vi "LiveAcquireold.vi"() -> ()   [LabVIEW 2015]
uses:
  <userlib>/atmcd64d.llb/AcquisitionMode_mode typedef.ctl
  NIDAQControls/StateGlobals.vi
  AcquisitionGlobals.vi
  NIDAQControls/NIDAQGlobals.vi
  LiveImage_Global.vi
panel:
  out "size(s)":i32
  out "xpixels 2":i32
  out "ypixels 2":i32
  out "Acquire Time":dbl
  out "Wait Time":dbl
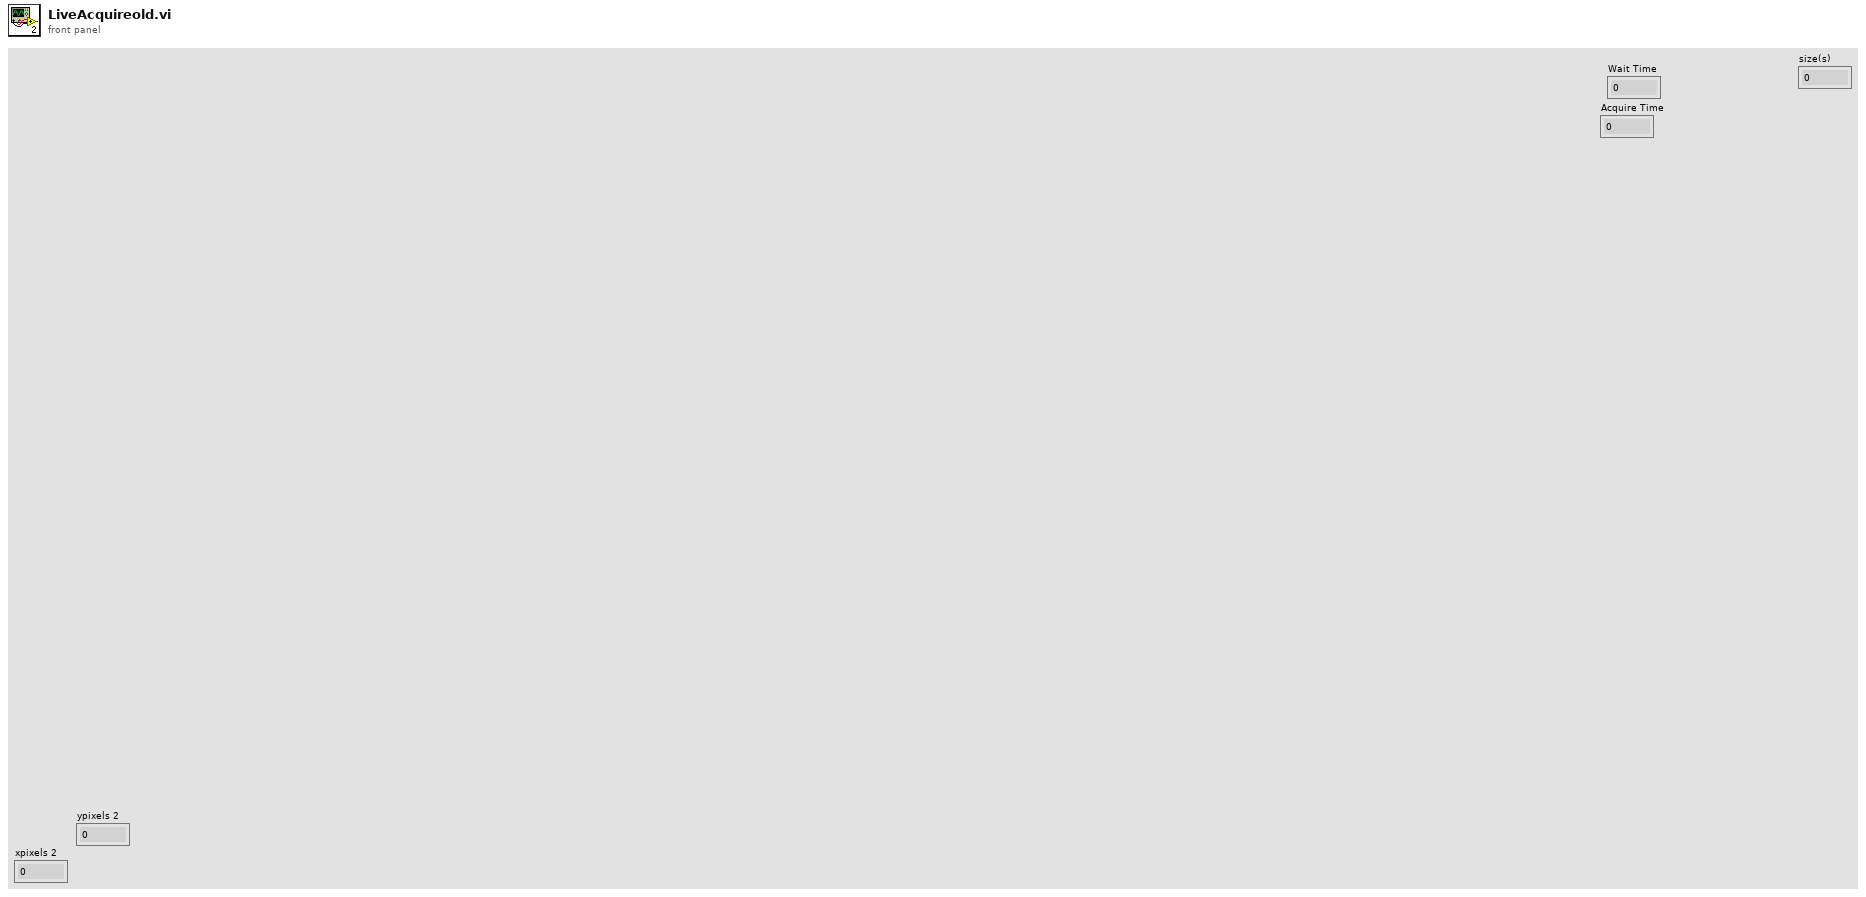
[diagram p1: front panel]
types:
  T1 = cluster{"Start or New Parameters?":bool, "Laser Mode":string, "Piezo Mode":string, "Begin Or End Acquisition":string, "Acquisition Time":dbl}
  T2 = typedef "AcquisitionMode_mode typedef.ctl" = enum16{"Reserved (0)", "Single Scan", "Accumulate", "Kinetics", "Fast Kinetics", "Run Till Abort", "Reserved (6)", "Reserved (7)", "Reserved (8)", "Time Delayed Integration"}
  T3 = typedef "Rendezvous RefNum" = refnum<k1>
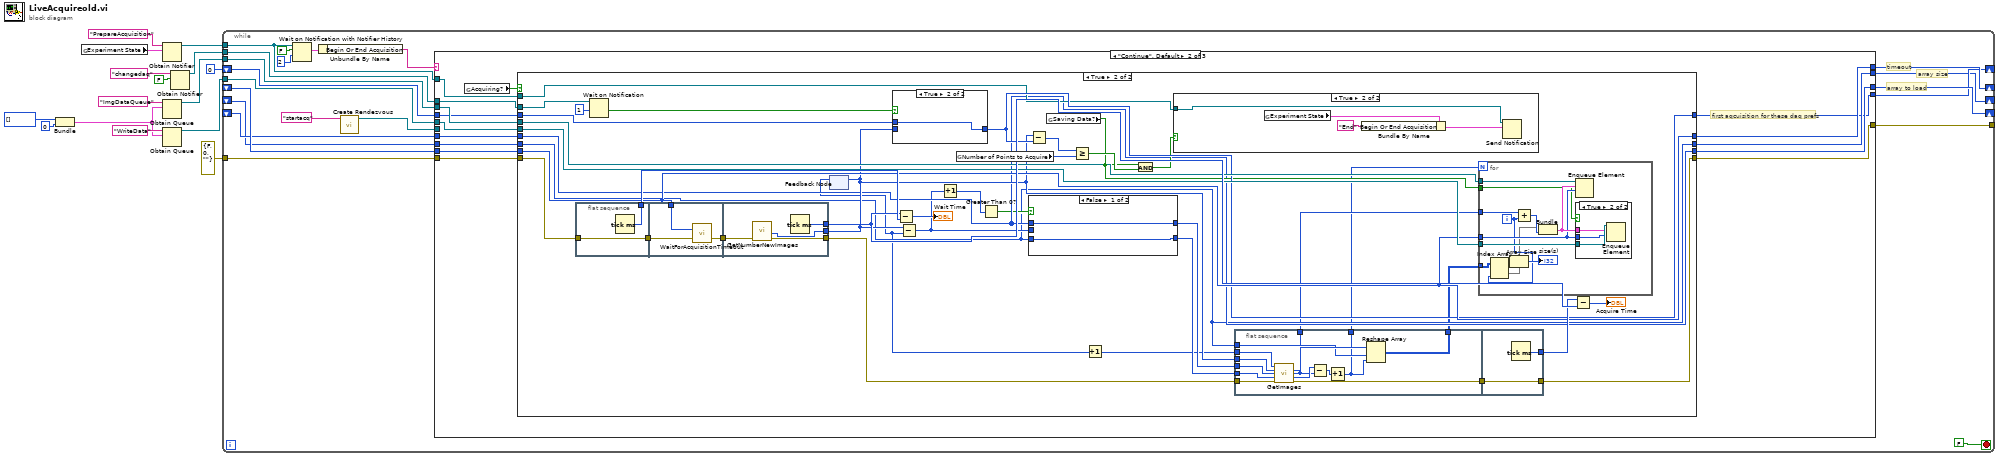
[diagram p0: block diagram]
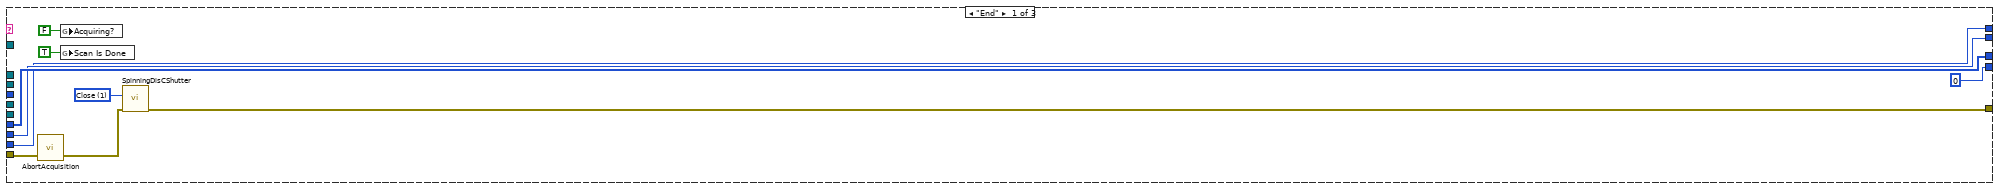
[diagram p2: hidden frame]
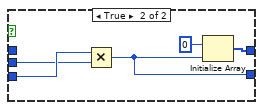
[diagram p5: hidden frame]
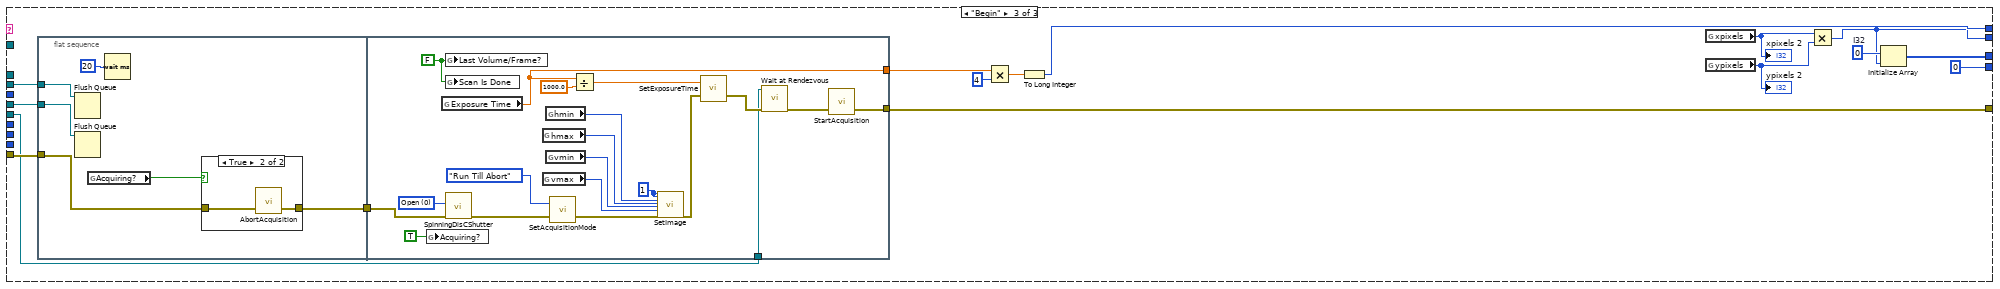
[diagram p8: hidden frame]
diagram:
  n1 = Bundle(u16[] [], 0) -> (w8:cluster{u16[], i32})  [unwired: 1 in]
  n2 = global read "StateGlobals.vi" "Experiment State"() -> (w1:T1)
  n3 = Obtain Notifier(name (unnamed)="PrepareAcquisition", notification data type=w1) -> (notifier out=w13:refnum<notifier>)  [unwired: 2 in, 2 out]
  n4 = Obtain Queue(name (unnamed)="ImgDataQueue", element data type=w8) -> (queue out=w6:refnum<queue>)  [unwired: 3 in, 2 out]
  n5 = Obtain Queue(name (unnamed)="WriteData", element data type=w8) -> (queue out=w7:refnum<queue>)  [unwired: 3 in, 2 out]
  n6 = Obtain Notifier(name (unnamed)="changedaq", notification data type=FALSE) -> (notifier out=w2:refnum<notifier>)  [unwired: 2 in, 2 out]
  n7 = while {
    tunnel: w13 -> [w17]
    shift-right: [w33] -> _
    shift-left: _ -> [w29]
    shift-right: [w32] -> _
    shift-left: _ -> [w28]
    shift-right: [w16] -> _
    shift-left: _ -> [w24]
    tunnel: w7 -> [w27]
    tunnel: w6 -> [w26]
    tunnel: errorcluster {"status"=FALSE, "code"=0, "source"=""} ("error out") -> [w31]
    tunnel: [w30] -> _
    shift-right: [w19] -> _
    shift-left: 0 -> [w20]
    tunnel: w2 -> [w18]
    stop <- FALSE stop-if-true
    # "array size"
    # "timeout"
    # "array to load"
    n8 = Wait on Notification with Notifier History(0:w17, 1:FALSE ("ignore previous (F)"), 2:2 ("timeout in ms (-1)")) -> (9:w35:T1)  [unwired: 1 in, 3 out]
    n9 = Unbundle By Name(w35) -> ("Begin Or End Acquisition"=w34:string)
    n10 = call <vilib>:"Create Rendezvous.vi"("name (unnamed)"="startacq") -> ("rendezvous"=w22:T3)  [unwired: 4 in, 2 out]
    n11 = case shown="\"Continue\", Default" w34 {
      tunnel: [w38 w54 w166] -> w33
      tunnel: [w40 w55 w165] -> w32
      tunnel: [w39 w53 w164] -> w16
      tunnel: w31 -> [w42 w59 w163]
      tunnel: [w41 w56 w162] -> w30
      tunnel: w29 -> [w38 w60 _]
      tunnel: w28 -> [w40 w58 _]
      tunnel: w24 -> [w39 w57 _]
      tunnel: w27 -> [_ w52 w157]
      tunnel: w26 -> [_ w51 w158]
      tunnel: w22 -> [_ _ w159]
      tunnel: w20 -> [_ w50 _]
      tunnel: [0 ("last") w48 0 ("last")] -> w19
      tunnel: w18 -> [_ w49 _]
      tunnel: w17 -> [_ w47 _]
      frame "End" {
        w44 = u16 1 items=["Open", "Close"] ("Ring")
        n12 = call <userlib>:"AbortAcquisition.vi"("error in (no error)"=w42) -> ("error out"=w43:errorcluster)  [unwired: 1 in, 1 out]
        n13 = global write "AcquisitionGlobals.vi" "Acquiring?"(FALSE) -> ()
        n14 = global write "NIDAQGlobals.vi" "Scan Is Done"(TRUE ("Last Volume/Frame?")) -> ()
        n15 = call "SpinningDisCShutter.vi"("error in (no error)"=w43, "Ring"=w44) -> ("error out"=w41:errorcluster)  [unwired: 9 in]
      }
      frame "Continue", Default {
        # "first aqcuisition for these daq prefs"
        n16 = global read "AcquisitionGlobals.vi" "Acquiring?"() -> (w61:bool)
        n17 = case shown="True" w61 {
          tunnel: w60 -> [w63 w91]
          tunnel: w59 -> [w65 w102]
          tunnel: w58 -> [w64 w78]
          tunnel: w57 -> [w66 w73]
          tunnel: [w65 w94] -> w56
          tunnel: [w64 w78] -> w55
          tunnel: [w63 w91] -> w54
          tunnel: [w66 w73] -> w53
          tunnel: w52 -> [_ w92]
          tunnel: w51 -> [_ w93]
          tunnel: w50 -> [w62 w88]
          tunnel: [w62 w87] -> w48
          tunnel: w49 -> [_ w90]
          tunnel: w47 -> [_ w82]
          frame False {
          }
          frame True {
            n18 = flat-sequence {
              tunnel: w102 -> [w148]
              tunnel: [w148] -> w104
              tunnel: [w147] -> w99
              tunnel: w104 -> [w151]
              tunnel: [w150] -> w103
              tunnel: w91 -> [w149]
              tunnel: [w153] -> w100
              tunnel: w103 -> [w154]
              tunnel: [w155] -> w97
              tunnel: [w152] -> w79
              frame #0 {
                n19 = Tick Count (ms)() -> (millisecond timer value=w147:u32)
              }
              frame #1 {
                n20 = call <userlib>:"WaitForAcquisitionTimeout.vi"("error in (no error)"=w151, "iTimeOutMs"=w149) -> ("error out"=w150:errorcluster)  [unwired: 1 out]
              }
              frame #2 {
                n21 = call <userlib>:"GetNumberNewImages.vi"("error in (no error)"=w154) -> ("error out"=w153:errorcluster, "last"=w152:i32)  [unwired: 3 in, 2 out]
                n22 = Tick Count (ms)() -> (millisecond timer value=w155:u32)
              }
            }
            n23 = Wait on Notification(notifier=w90, timeout in ms (-1)=1) -> (timed out?=w89:bool)  [unwired: 2 in, 3 out]
            n24 = feedback-in #1(w79) -> ()
            n25 = feedback #1() -> (w68:i32)  [unwired: 1 in]
            n26 = case shown="True" w89 {
              tunnel: w88 -> [_ w131]
              tunnel: w79 -> [w130 _]
              tunnel: [w130 w131] -> w87
              frame False {
              }
              frame True {
              }
            }
            n27 = Subtract(x=w97, y=w99) -> (x-y=→"Wait Time":u32)
            n28 = Subtract(x=w79, y=w68) -> (x-y=w74:i32)
            n29 = Increment(x=w74) -> (x+1=w70:i32)
            n30 = global read "StateGlobals.vi" "Number of Points to Acquire"() -> (w85:i32)
            n31 = Greater Than 0?(x=w70) -> (x > 0?=w75:bool)
            n32 = case shown="False" w75 {
              tunnel: w73 -> [w119 w124]
              tunnel: w78 -> [w120 _]
              tunnel: [w120 w122] -> w77
              tunnel: [w119 w121] -> w76
              tunnel: w74 -> [_ w123]
              frame False {
              }
              frame True {
                n33 = Multiply(x=w124, y=w123) -> (x*y=w121:i32)
                n34 = Initialize Array(u16 0 ("element"), w121) -> (w122:u16[])
              }
            }
            n35 = Subtract(x=w79, y=w87) -> (x-y=w80:i32)
            n36 = global read "AcquisitionGlobals.vi" "Saving Data?"() -> (w83:bool)
            n37 = Greater Or Equal?(x=w80, y=w85) -> (x >= y?=w84:bool)
            n38 = Increment(x=w68) -> (x+1=w69:i32)
            n39 = And(x=w83, y=w84) -> (x .and. y?=w81:bool)
            n40 = case shown="True" w81 {
              tunnel: w82 -> [_ w129]
              frame False {
              }
              frame True {
                n41 = global read "StateGlobals.vi" "Experiment State"() -> (w128:T1)
                n42 = Bundle By Name(cluster=w128, "Begin Or End Acquisition"="End") -> (w126:T1)
                n43 = Send Notification(notification=w126, notifier=w129) -> ()  [unwired: 1 in, 2 out]
              }
            }
            n44 = flat-sequence {
              tunnel: w77 -> [w140]
              tunnel: [w144] -> w101
              tunnel: w100 -> [w143]
              tunnel: w79 -> [w142]
              tunnel: w69 -> [w141]
              tunnel: w76 -> [w139]
              tunnel: w73 -> [w136]
              tunnel: [w135] -> w72
              tunnel: [w134] -> w71
              tunnel: [w132] -> w67
              tunnel: [w146] -> w94
              tunnel: w101 -> [w146]
              tunnel: [w145] -> w96
              frame #0 {
                n45 = call <userlib>:"GetImages.vi"("first"=w141, "last"=w142, "array"=w140, "size"=w139, "error in (no error)"=w143) -> ("array"=w138:i32[], "validfirst"=w134:i32, "validlast"=w137:i32, "error out"=w144:errorcluster)  [unwired: 6 in, 1 out]
                n46 = Subtract(x=w137, y=w134) -> (x-y=w133:i32)
                n47 = Increment(x=w133) -> (x+1=w132:i32)
                n48 = Reshape Array(w138, w136, w132) -> (w135:i32[][])
              }
              frame #1 {
                n49 = Tick Count (ms)() -> (millisecond timer value=w145:u32)
              }
            }
            n50 = for {
              N: w67 -> [_]
              tunnel: w93 -> [w114]
              tunnel: w92 -> [w113]
              tunnel: w91 -> [w112]
              tunnel: w83 -> [w111]
              tunnel: w72 -> [w107]
              tunnel: w71 -> [w110]
              i -> [w106]
              n51 = Index Array(array=w107, index (col)=w106) -> (element=w105:i32[])  [unwired: 1 in]
              n52 = Array Size(array=w105) -> (size(s)=→"size(s)":i32)
              n53 = Add(x=w110, y=w106) -> (x+y=w109:i32)
              n54 = Bundle("array"=w105, w109) -> (w115:cluster{"array":i32[], i32})  [unwired: 1 in]
              n55 = Enqueue Element(queue=w114, element=w115, timeout in ms (-1)=w112) -> ()  [unwired: 1 in, 3 out]
              n56 = case shown="True" w111 {
                tunnel: w113 -> [_ w118]
                tunnel: w112 -> [_ w117]
                tunnel: w115 -> [_ w116]
                frame False {
                }
                frame True {
                  n57 = Enqueue Element(queue=w118, element=w116, timeout in ms (-1)=w117) -> ()  [unwired: 1 in, 3 out]
                }
              }
            }
            n58 = Subtract(x=w96, y=w97) -> (x-y=→"Acquire Time":u32)
          }
        }
      }
      frame "Begin" {
        w169 = u16 0  # I32
        n59 = flat-sequence {
          tunnel: w163 -> [w177]
          tunnel: [w176] -> w161
          tunnel: w158 -> [w174]
          tunnel: w157 -> [w173]
          tunnel: [w196] -> w162
          tunnel: w161 -> [w197]
          tunnel: [w184] -> w160
          tunnel: w159 -> [w181]
          frame #0 {
            n60 = Flush Queue(queue=w174) -> ()  [unwired: 1 in, 3 out]
            n61 = Flush Queue(queue=w173) -> ()  [unwired: 1 in, 3 out]
            n62 = global read "AcquisitionGlobals.vi" "Acquiring?"() -> (w175:bool)
            n63 = Wait (ms)(milliseconds to wait=u32 20) -> ()  [unwired: 1 out]
            n64 = case shown="True" w175 {
              tunnel: w177 -> [w178 w180]
              tunnel: [w178 w179] -> w176
              frame False {
              }
              frame True {
                n65 = call <userlib>:"AbortAcquisition.vi"("error in (no error)"=w180) -> ("error out"=w179:errorcluster)  [unwired: 1 in, 1 out]
              }
            }
          }
          frame #1 {
            w193 = 1
            w195 = FALSE ("Last Volume/Frame?")
            w199 = u16 0 items=["Open", "Close"] ("Ring")
            n66 = global write "AcquisitionGlobals.vi" "Acquiring?"(TRUE) -> ()
            n67 = global read "LiveImage_Global.vi" "Exposure Time"() -> (w184:dbl)
            n68 = global write "NIDAQGlobals.vi" "Last Volume/Frame?"(w195) -> ()
            n69 = global write "NIDAQGlobals.vi" "Scan Is Done"(w195) -> ()
            n70 = call "SpinningDisCShutter.vi"("error in (no error)"=w197, "Ring"=w199) -> ("error out"=w198:errorcluster)  [unwired: 9 in]
            n71 = global read "LiveImage_Global.vi" "hmax"() -> (w191:i32)
            n72 = global read "LiveImage_Global.vi" "vmax"() -> (w189:i32)
            n73 = global read "LiveImage_Global.vi" "hmin"() -> (w192:i32)
            n74 = global read "LiveImage_Global.vi" "vmin"() -> (w190:i32)
            n75 = call <userlib>:"SetAcquisitionMode.vi"("error in (no error)"=w198, "mode"=AcquisitionMode_mode_typedef."Run Till Abort") -> ("error out"=w188:errorcluster)  [unwired: 1 out]
            n76 = Divide(x=w184, y=1000.0) -> (x/y=w185:dbl)
            n77 = call <userlib>:"SetImage.vi"("hbin"=w193, "vbin"=w193, "hstart"=w192, "hend"=w191, "vstart"=w190, "vend"=w189, "error in (no error)"=w188) -> ("error out"=w187:errorcluster)  [unwired: 19 in, 1 out]
            n78 = call <userlib>:"SetExposureTime.vi"("error in (no error)"=w187, "time"=w185) -> ("error out"=w183:errorcluster)  [unwired: 1 out]
            n79 = call <vilib>:"Wait at Rendezvous.vi"("error in (no error)"=w183, "rendezvous"=w181) -> ("error out"=w182:errorcluster)  [unwired: 3 in, 2 out]
            n80 = call <userlib>:"StartAcquisition.vi"("error in (no error)"=w182) -> ("error out"=w196:errorcluster)  [unwired: 1 in, 1 out]
          }
        }
        n81 = Multiply(x=w160, y=4) -> (x*y=w167:dbl)
        n82 = To Long Integer(number=w167) -> (32bit integer=w166:i32)
        n83 = global read "LiveImage_Global.vi" "xpixels"() -> (w170:i32)
        "xpixels 2" <- w170
        n84 = global read "LiveImage_Global.vi" "ypixels"() -> (w171:i32)
        "ypixels 2" <- w171
        n85 = Multiply(x=w170, y=w171) -> (x*y=w164:i32)
        n86 = Initialize Array "Initialize Array"(w169, w164) -> (w165:u16[])
      }
    }
  }
